vi "Data Source Add Group.vi"(11 "Data In":string[](array[string])) -> (1 "Name":string, 2 "OK？":bool, 3 "Data Out":string[](array[string]))   [LabVIEW 2020]
panel:
  in  "Cancle":bool
  in  "OK":bool
  in  "Use":bool
  in  "Name In":string caption="名称"
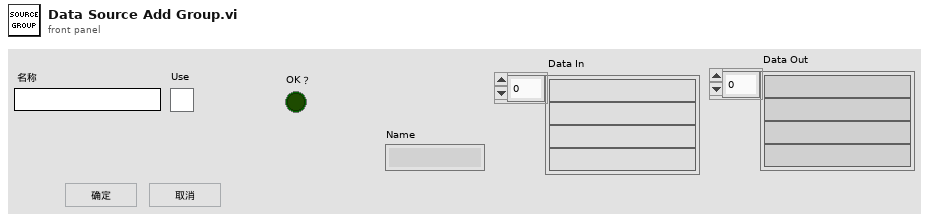
[diagram p1: front panel]
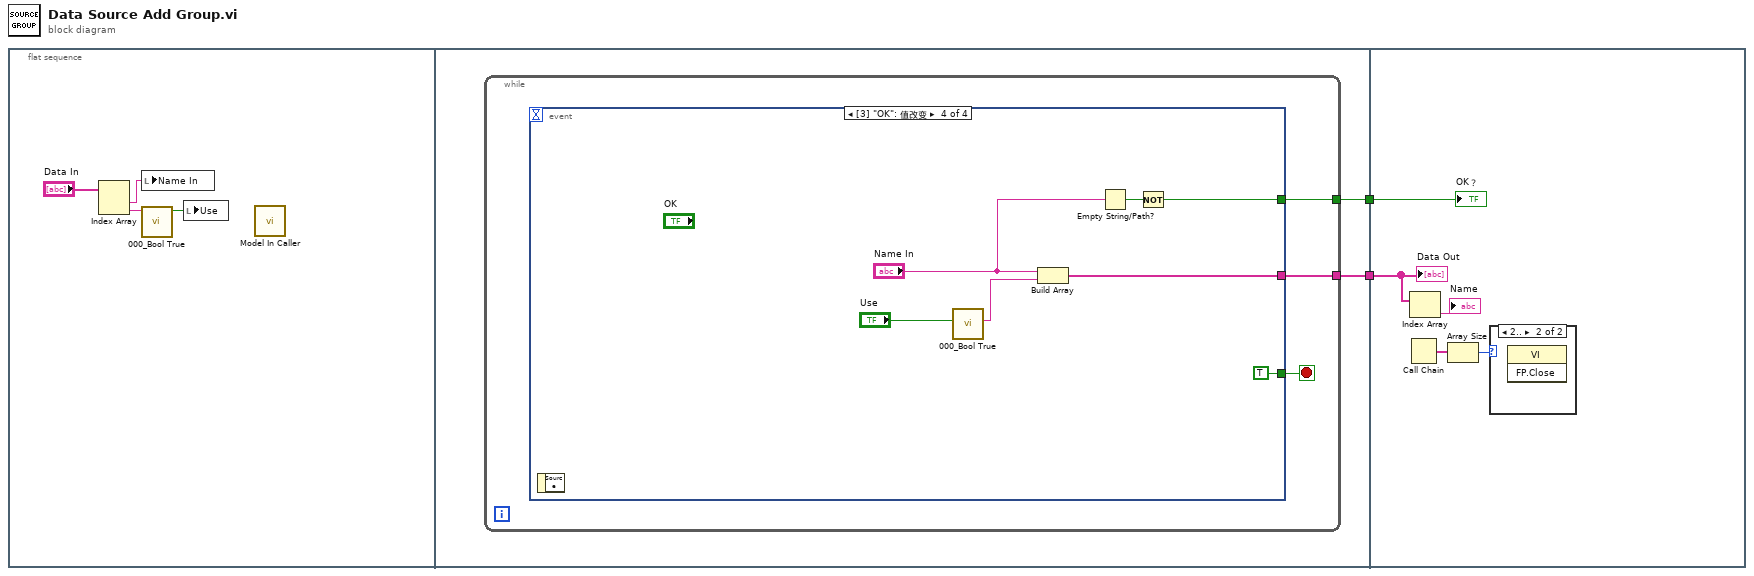
[diagram p0: block diagram]
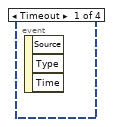
[diagram p2: hidden frame]
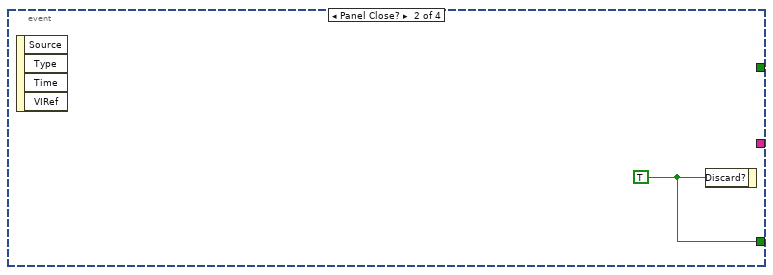
[diagram p3: hidden frame]
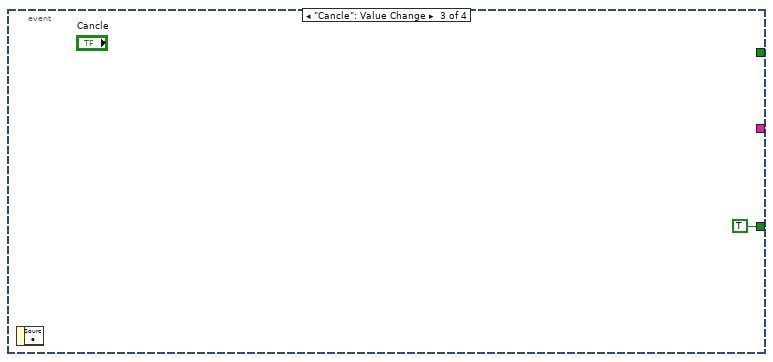
[diagram p4: hidden frame]
diagram:
  n1 = flat-sequence {
    tunnel: [w8] -> w2
    tunnel: [w7] -> w1
    tunnel: w2 -> [w25]
    tunnel: w1 -> [w22]
    frame #0 {
      n2 = Index Array(array="Data In") -> (element #1=w5:string, element #2=w4:string)  [unwired: 2 in]
      n3 = local write "Name In"(w5) -> ()
      n4 = call "000_Bool True.vi"("Bool String"=w4) -> ("True"=w3:bool)  [unwired: 8 in, 2 out]
      n5 = local write "Use"(w3) -> ()
      n6 = call "Model In Caller.vi"() -> ()  [unwired: 11 in, 1 out]
    }
    frame #1 {
      n7 = while {
        tunnel: [w10] -> w8
        tunnel: [w9] -> w7
        stop <- w11 stop-if-true
        n8 = event shown="[3] \"OK\": 值改变" {
          selector: _ -> [_ _ _ _]
          dyn-events: _ -> [_ _ _ _]
          timeout: _ -> [_ _ _ _]
          tunnel: [_ w12 TRUE ("放弃？") TRUE ("放弃？")] -> w11
          tunnel: [_ _ _ w14] -> w10
          tunnel: [_ _ _ w17] -> w9
          event Timeout {
            n9 = event-data() -> ()  [unwired: 1 in, 3 out]
          }
          event Panel Close? {
            w12 = TRUE ("放弃？")
            n10 = event-data() -> ()  [unwired: 1 in, 4 out]
            n11 = event-data("Discard?"=w12) -> ()  [unwired: 1 in, 1 out]
          }
          event "Cancle": Value Change {
            n12 = event-data() -> ()  [unwired: 1 in, 1 out]
          }
          event "OK": Value Change {
            n13 = event-data() -> ()  [unwired: 1 in, 1 out]
            n14 = call "000_Bool True.vi"("Value"="Use") -> ("String Out"=w18:string)  [unwired: 8 in, 2 out]
            n15 = Build Array("Name In", w18) -> (w17:string[])
            n16 = Empty String/Path?(string/path="Name In") -> (empty?=w15:bool)
            n17 = Not(x=w15) -> (.not. x?=w14:bool)
          }
        }
      }
    }
    frame #2 {
      n18 = Call Chain() -> (call chain=w24:string[])
      n19 = Index Array(array=w22) -> (element=→"Name":string)  [unwired: 1 in]
      n20 = Array Size(array=w24) -> (size(s)=w23:i32)
      n21 = case shown="2.." w23 {
        frame 0, Default {
        }
        frame 2.. {
          n22 = invoke class="VI" method="FP.Close"() -> ()  [unwired: 3 in, 3 out]
        }
      }
      "OK？" <- w25
      "Data Out" <- w22
    }
  }
